vi "ADD Script.vi"(8 "error in (no error)":errorcluster, 11 "Comando":string) -> (0 "error out":errorcluster, 3 "Comando RTS":string)   [LabVIEW 2014, in "CAP-USB.lvlib"]
doc: "Genera el codigo para agregar una script\nal CAP-USB"
uses:
  CAP-USB.lvlib
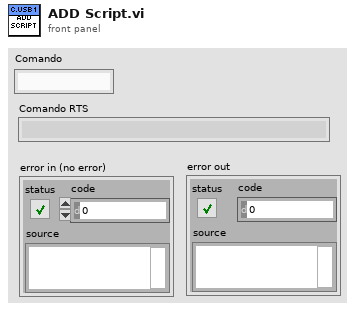
[diagram p1: front panel]
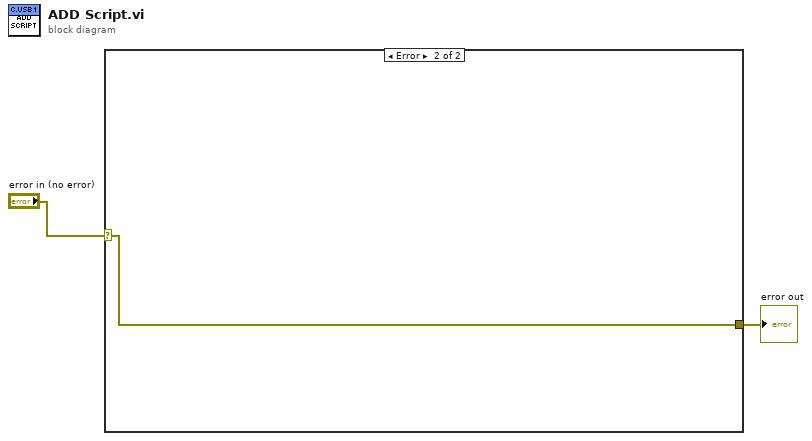
[diagram p0: block diagram]
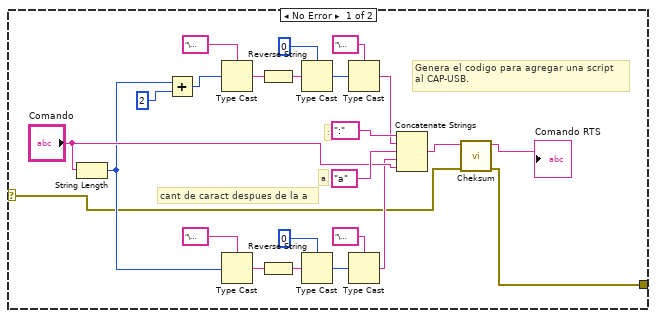
[diagram p2: hidden frame]
diagram:
  n1 = case shown="Error" "error in (no error)" {
    selector: "error in (no error)" -> [w4 w27]
    tunnel: [w3 w27] -> w1
    frame No Error {
      # "Genera el codigo para agregar una script\nal CAP-USB."
      # "cant de caract despues de la a"
      # "a"
      # ":"
      n2 = String Length(string="Comando") -> (length=w8:i32)
      n3 = Add(x=w8, y=2) -> (x+y=w22:i32)
      n4 = Type Cast(type="\u0000" ("string"), x=w22) -> (*(type *) &x=w19:string)
      n5 = Type Cast(type="\u0000" ("string"), x=w8) -> (*(type *) &x=w11:string)
      n6 = Reverse String(1:w19) -> (0:w18:string)
      n7 = Reverse String(1:w11) -> (0:w12:string)
      n8 = Type Cast(type=u8 0 ("y"), x=w18) -> (*(type *) &x=w16:u8)
      n9 = Type Cast(type=u8 0 ("y"), x=w12) -> (*(type *) &x=w14:u8)
      n10 = Type Cast(type="\u0000" ("string"), x=w16) -> (*(type *) &x=w15:string)
      n11 = Type Cast(type="\u0000" ("string"), x=w14) -> (*(type *) &x=w7:string)
      n12 = Concatenate Strings(":" ("string"), w15, "a" ("string"), w7, "Comando") -> (w5:string)
      n13 = call "Cheksum.vi"("error in (no error)"=w4, "Trama IN"=w5) -> ("error out"=w3:errorcluster, "Trama RTS"=→"Comando RTS":string)  [unwired: 8 in]
    }
    frame Error {
    }
  }
  "error out" <- w1
